vi "Auto-Refresh Read.vi"(8 "error in (no error)":errorcluster, 11 "MSX-E3701 in":refnum<class "MSX-E3701.lvclass">) -> (0 "error out":errorcluster, 1 "Control Data":T1, 2 "1 Sample":T2, 3 "MSX-E3701 out":refnum<class "MSX-E3701.lvclass">)   [LabVIEW 2014, in "MSX-E3701.lvlib" / "MSX-E3701.lvclass"]
doc: "Inicia la lectura de datos y los afecta a estos con la ganancia y el offset que previamente se configuraron."
uses:
  MSX-E3701.lvclass
  DriverMasterSync/build/DriverMasterSync.lvlibp/APIs/Data Queue/Acquisition Data 1 Sample Cluster.ctl
  DriverMasterSync/build/DriverMasterSync.lvlibp/APIs/Data Queue/Control Data Cluster.ctl
  MSX-E3701.lvclass/MSX-E3701.ctl
  DriverMasterSync/build/DriverMasterSync.lvlibp/Modules/HAL/DriverMasterSync/DriverMasterSyncClass/DriverMasterSync.lvclass
  API/MSX-E3701_dll.lvlib
  DriverMasterSync/build/DriverMasterSync.lvlibp/APIs/Data Queue/WINFAS 2 Data Queue.lvlib
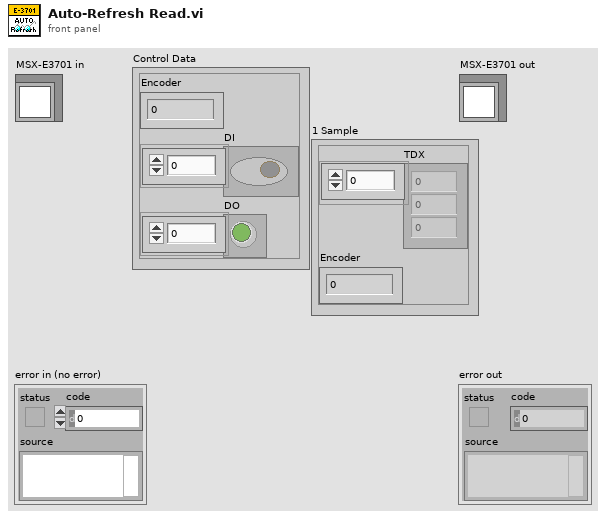
[diagram p1: front panel]
types:
  T1 = typedef "DriverMasterSync.lvlibp/WINFAS 2 Data Queue.lvlib/Control Data Cluster.ctl" = cluster{"Encoder":sgl, "DI":bool[], "DO":bool[]}
  T2 = typedef "DriverMasterSync.lvlibp/WINFAS 2 Data Queue.lvlib/Acquisition Data 1 Sample Cluster.ctl" = cluster{"TDX":sgl[], "Encoder":sgl}
  T3 = typedef "MSX-E3701_dll.lvlib/Connection Data.ctl" = cluster{"MX370x refnum":refnum<k24>, "IP":string, "Connection ID ":refnum<k5>, "MXCommon refnum":refnum<k24>}
  T4 = typedef "MSX-E3701_dll.lvlib/Adquisition Data.ctl" = cluster{"Adq. Sequence":cluster{"TSs - TSu - NAS":u64[][], "Adquisition Value":u32[][], "Status IO Port":bool[]}, "Adq. Auto Refresh":cluster{"Adquisition Value":u64[], "Status IO Port":bool[], "Counter value":u64[]}}
  T5 = cluster{"Adquisition Value":u64[], "Status IO Port":bool[], "Counter value":u64[]}
  T6 = typedef "DriverMasterSync.lvlibp/HAL Config Data.ctl" = cluster{"HWSync Index":u32, "Driver Name":string, "Channel Mask":u64}
  T7 = typedef "DriverMasterSync.lvlibp/WINFAS 2 Data Queue.lvlib/Acquisition Data Cluster.ctl" = T2[]
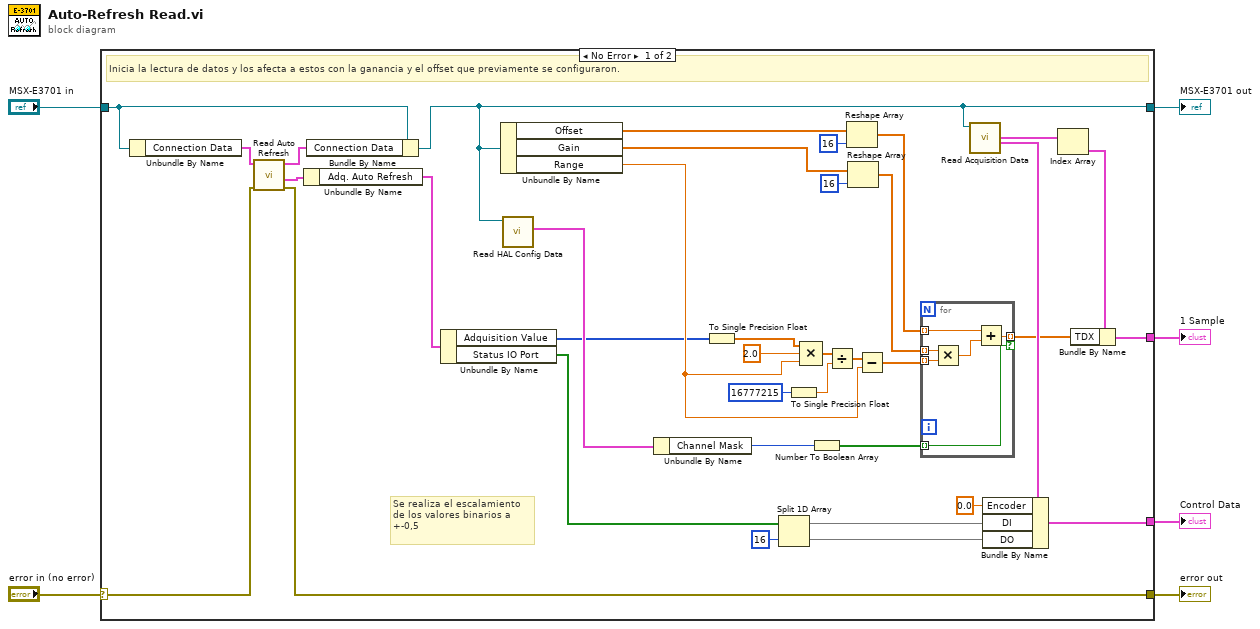
[diagram p0: block diagram]
diagram:
  n1 = case shown="No Error" "error in (no error)" {
    selector: "error in (no error)" -> [w30 w51]
    tunnel: [w16 w51] -> w5
    tunnel: [w22 w50] -> w3
    tunnel: "MSX-E3701 in" -> [w31 w50]
    tunnel: [w29 _] -> w1
    tunnel: [w18 _] -> w2
    frame No Error {
      # "Se realiza el escalamiento de los valores binarios a \n+-0,5"
      # "Inicia la lectura de datos y los afecta a estos con la ganancia y el offset que previamente se configuraron."
      n2 = Unbundle By Name(w31) -> ("Connection Data"=w43:T3)
      n3 = call "Read Auto Refresh.vi"("error in (no error)"=w30, "Connection Data In"=w43) -> ("error out"=w16:errorcluster, "Adquisition Data Out"=w42:T4, "Connection Data Out"=w33:T3)  [unwired: 7 in]
      n4 = Unbundle By Name(w42) -> ("Adq. Auto Refresh"=w38:T5)
      n5 = Bundle By Name(cluster=w31, "Connection Data"=w33) -> (w22:refnum<class "MSX-E3701.lvclass">)
      n6 = Unbundle By Name(w38) -> ("Adquisition Value"=w7:u64[], "Status IO Port"=w37:bool[])
      n7 = Unbundle By Name(w22) -> ("Offset"=w28:sgl[], "Gain"=w25:sgl[], "Range"=w9:sgl)
      n8 = call "Read HAL Config Data.vi"("DriverMasterSync in"=w22) -> ("HAL Config Data"=w21:T6)  [unwired: 8 in, 2 out]
      n9 = Unbundle By Name(w21) -> ("Channel Mask"=w20:u64)
      n10 = To Single Precision Float(number=w7) -> (single precision float=w13:sgl[])
      n11 = Split 1D Array(array=w37, index=16) -> (first subarray=w36:bool[], second subarray=w35:bool[])
      n12 = To Single Precision Float(number=u64 16777215 ("x")) -> (single precision float=w14:sgl)
      n13 = Compound Arithmetic op=MULTIPLY(w13, sgl 2.0 ("x"), w9) -> (w12:sgl[])
      n14 = Number To Boolean Array(number=w20) -> (Boolean array=w19:bool[])
      n15 = Divide(x=w12, y=w14) -> (x/y=w11:sgl[])
      n16 = Reshape Array(w28, 16 ("dimension size")) -> (w23:sgl[])
      n17 = Reshape Array(w25, 16 ("dimension size")) -> (w24:sgl[])
      n18 = Subtract(x=w11, y=w9) -> (x-y=w8:sgl[])
      n19 = for {
        tunnel: w24 -> [w49] mode=indexing
        tunnel: w23 -> [w48] mode=indexing
        tunnel: w8 -> [w46] mode=indexing
        tunnel: [w45] -> w17 mode=indexing if=w44
        tunnel: w19 -> [w44] mode=indexing
        n20 = Multiply(x=w49, y=w46) -> (x*y=w47:sgl)
        n21 = Add(x=w48, y=w47) -> (x+y=w45:sgl)
      }
      n22 = call "Read Acquisition Data.vi"("DriverMasterSync in"=w22) -> ("Control Data"=w39:T1, "Acquisition Data"=w41:T7)  [unwired: 7 in, 2 out]
      n23 = Bundle By Name(cluster=w39, "Encoder"=sgl 0.0, "DI"=w36, "DO"=w35) -> (w29:T1)
      n24 = Index Array(array=w41) -> (element=w40:T2)  [unwired: 1 in]
      n25 = Bundle By Name(cluster=w40, "TDX"=w17) -> (w18:T2)
    }
    frame Error {
    }
  }
  "error out" <- w5
  "MSX-E3701 out" <- w3
  "1 Sample" <- w2
  "Control Data" <- w1
